vi "Project Path--constant.vi"() -> (3 "Path":path=path "C:/GitClones/Unit Tests/yatzy-bug/yatzy refactoring.lvproj")   [LabVIEW 2024, in "Acquisition.lvlib"]
uses:
  Acquisition.lvlib
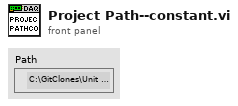
[diagram p1: front panel]
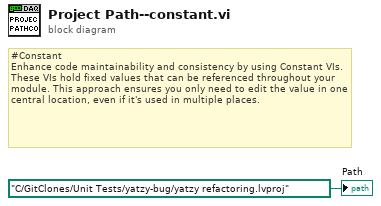
[diagram p0: block diagram]
diagram:
  # "#Constant\nEnhance code maintainability and consistency by using Constant VIs. These VIs hold fixed values that can be referenced throughout your module. This approach ensures you only need to edit the value in one central location, even if it's used in multiple places."
  "Path" <- path "C:/GitClones/Unit Tests/yatzy-bug/yatzy refactoring.lvproj" ("Path")
